vi "Apply configuration.vi"(8 "error in (no error)":errorcluster, 11 "CCD in":refnum<class "CCD.lvclass">) -> (0 "error out":errorcluster, 3 "CCD out":refnum<class "CCD.lvclass">)   [LabVIEW 2016, in "CCD.lvlib" / "CCD.lvclass"]
uses:
  <userlib>/Common Components/Hardware/CCD/CCD/CCD.lvclass
  <userlib>/Common Components/Hardware/CCD/CCD/CCD.lvclass/CCD.ctl
  <vilib>/vision/driver/NI_Vision_Acquisition_Software.lvlib
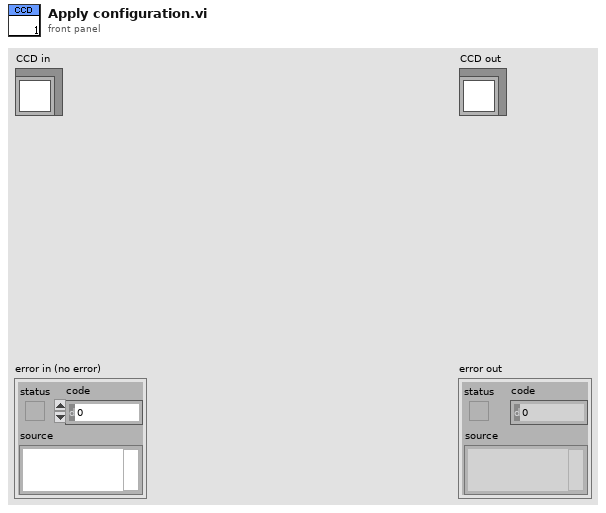
[diagram p1: front panel]
types:
  T1 = typedef "IMAQdx.ctl" = refnum<k21>
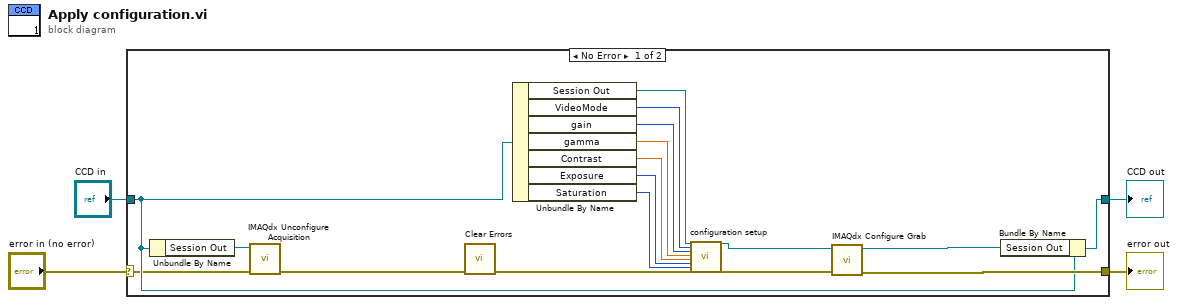
[diagram p0: block diagram]
diagram:
  n1 = case shown="No Error" "error in (no error)" {
    selector: "error in (no error)" -> [w7 w23]
    tunnel: [w10 w23] -> w3
    tunnel: [w12 w22] -> w1
    tunnel: "CCD in" -> [w9 w22]
    frame No Error {
      n2 = Unbundle By Name(w9) -> ("Session Out"=w8:T1)
      n3 = call <vilib>:"IMAQdx Unconfigure Acquisition.vi"("error in"=w7, "Session In"=w8) -> ("error out"=w6:errorcluster)  [unwired: 8 in, 1 out]
      n4 = call <vilib>:"Clear Errors.vi"("error in (no error)"=w6) -> ("error out"=w5:errorcluster)  [unwired: 5 in, 1 out]
      n5 = Unbundle By Name(w9) -> ("Session Out"=w21:T1, "VideoMode"=w20:u16, "gain"=w19:u32, "gamma"=w18:sgl, "Contrast"=w17:dbl, "Exposure"=w16:u32, "Saturation"=w15:u32)
      n6 = call <userlib>:"configuration setup.vi"("IMAQdx Session"=w21, "VideoMode"=w20, "Gain"=w19, "Gamma"=w18, "Contrast"=w17, "Exposure"=w16, "Saturation"=w15, "error in (no error)"=w5) -> ("IMAQdx Session 2"=w14:T1, "error out"=w11:errorcluster)  [unwired: 18 in]
      n7 = call <vilib>:"IMAQdx Configure Grab.vi"("error in"=w11, "Session In"=w14) -> ("error out"=w10:errorcluster, "Session Out"=w13:T1)  [unwired: 8 in]
      n8 = Bundle By Name(cluster=w9, "Session Out"=w13) -> (w12:refnum<class "CCD.lvclass">)
    }
    frame Error {
    }
  }
  "error out" <- w3
  "CCD out" <- w1
